vi "ArrayToSpreaSheet (SubVI).vi"(11 "ArrayTelemetryStr":string[][](array[string])) -> (3 "spreadsheet string":string)   [LabVIEW 2017]
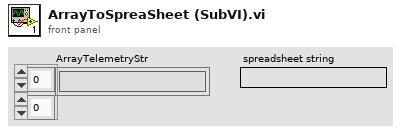
[diagram p1: front panel]
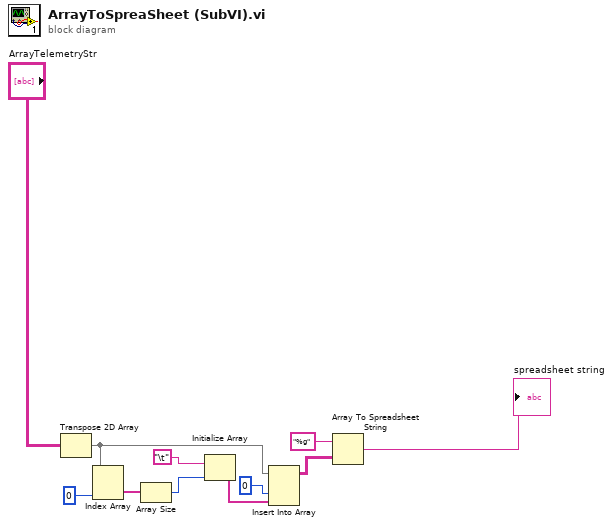
[diagram p0: block diagram]
diagram:
  n1 = Transpose 2D Array(2D array="ArrayTelemetryStr") -> (transposed array=w5:string[][])
  n2 = Index Array(array=w5, index (col)=0 ("disabled index (col)")) -> (element=w7:string[])  [unwired: 1 in]
  n3 = Array Size(array=w7) -> (size(s)=w8:i32)
  n4 = Initialize Array("\t", w8) -> (w11:string[])
  n5 = Insert Into Array(array=w5, index (col)=0 ("index (row)"), new element=w11) -> (w10:string[][])  [unwired: 1 in]
  n6 = Array To Spreadsheet String(array=w10, 3:"%g" ("format string")) -> (spreadsheet string=→"spreadsheet string":string)  [unwired: 1 in]
